vi "HEWH_VESTA_Main.vi"(6 "Vesta is working":refnum<vi>, 8 "error in":errorcluster, 11 "Message Queues out":T2) -> (0 "error out":errorcluster)   [LabVIEW 2023]
uses:
  Tenney/support/Message Queue/All Message Queues.ctl
  Tenney/support/Message Queue/Message Cluster.ctl
  Drivers/Resideo Gas Valve/Type Definitions/Vesta Info.ctl
  Drivers/Resideo Gas Valve/Type Definitions/Temperature Control.ctl
  FVIR and LDO/support/Message Queue/Enqueue Message (Single).vi
  FVIR and LDO/support/Message Queue/Message Queue.lvlib
  Tenney/support/Message Queue/Tenney Message Queue.lvlib
panel:
  out "Vesta Data Output":T1
  out "Debug":string[](array[string])
  in  "Debug":bool
  out "Loop Count":i32
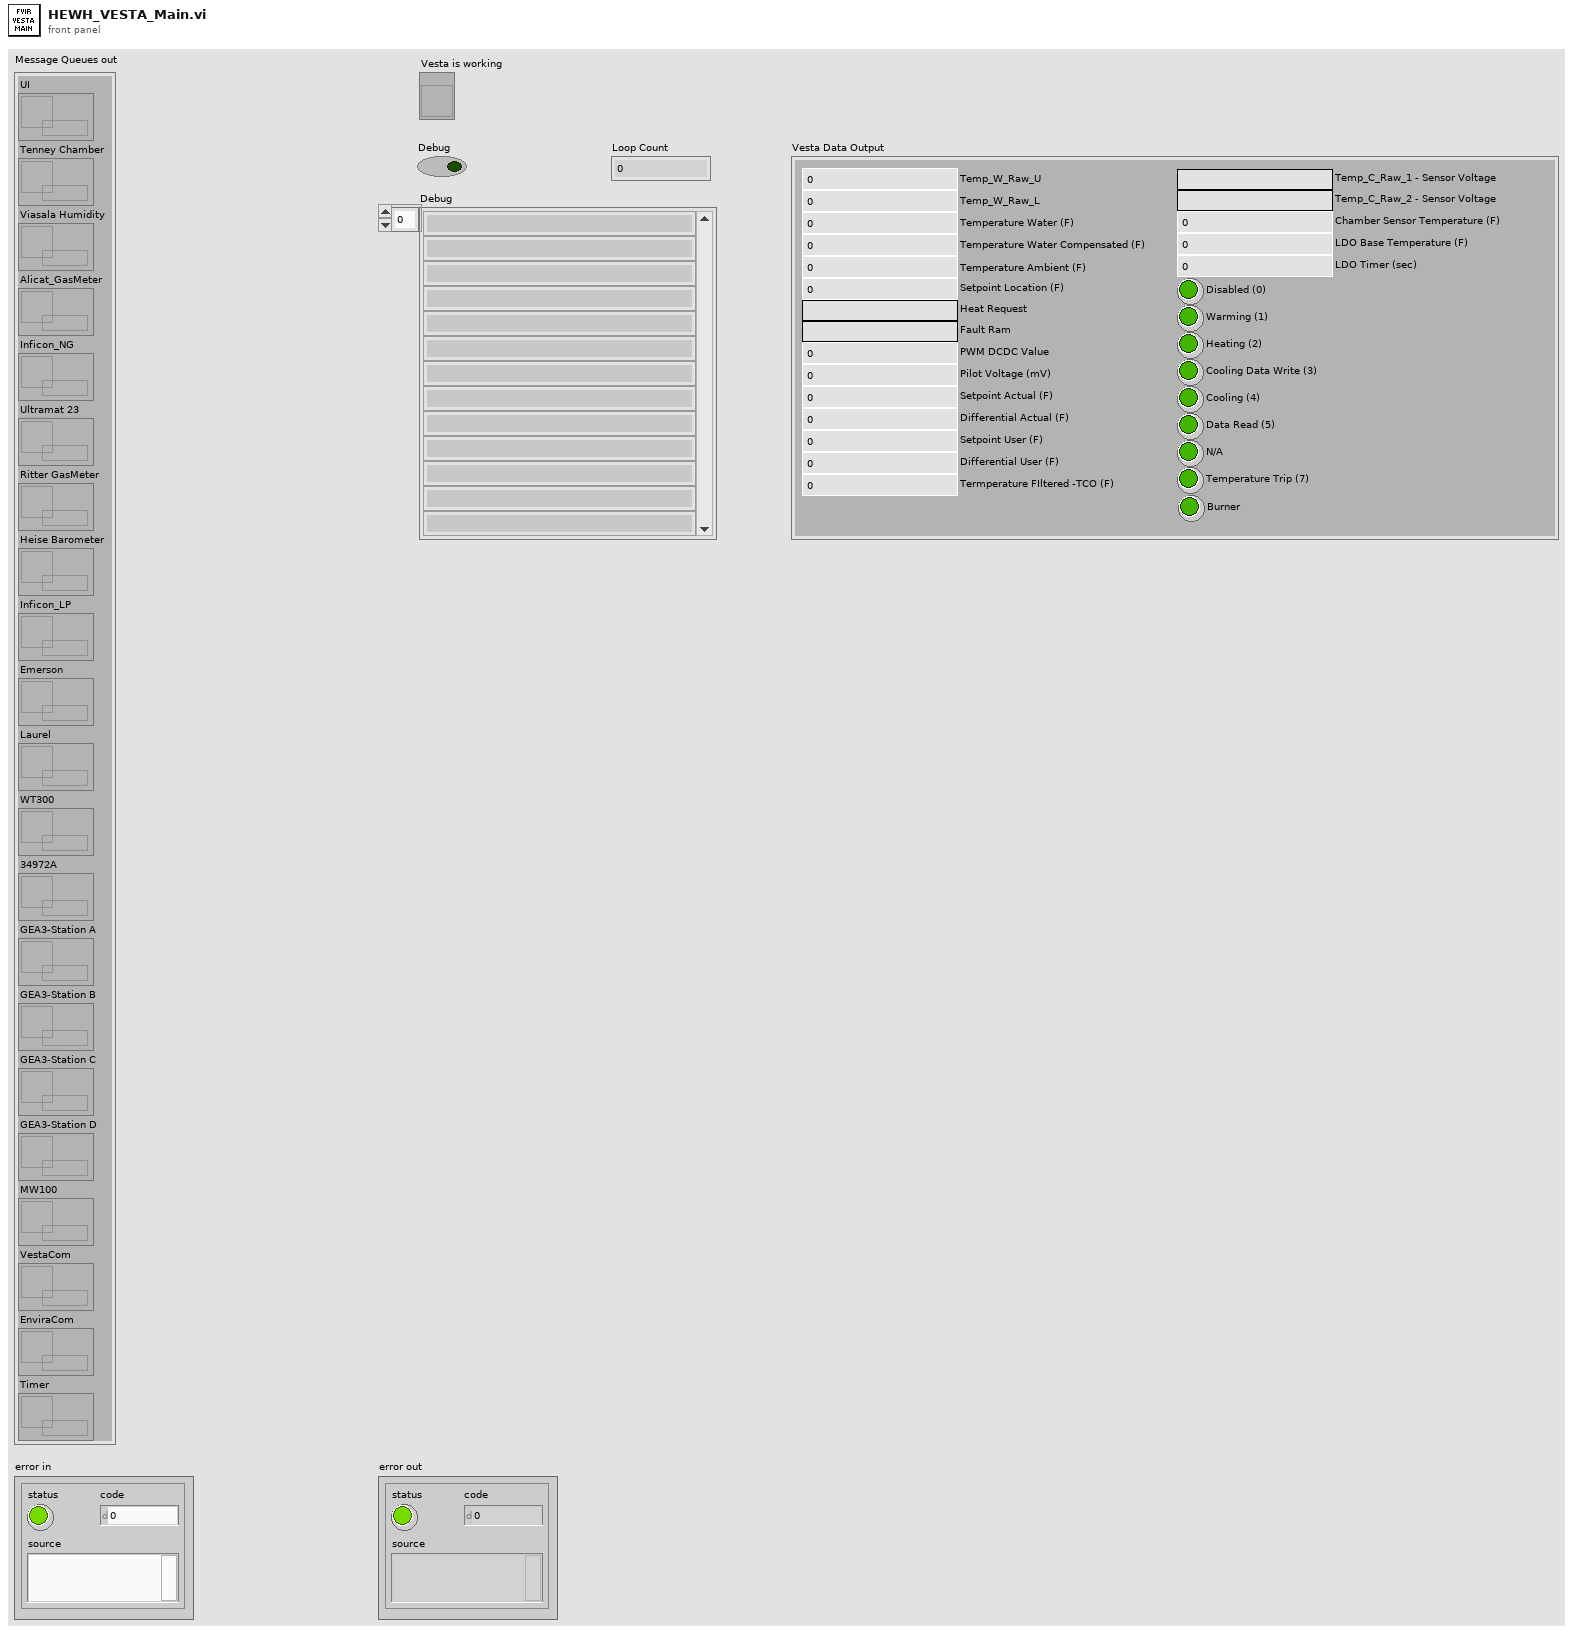
[diagram p1: front panel]
types:
  T1 = typedef "Vesta Info.ctl" = cluster{"Temp_W_Raw_U":u16, "Temp_W_Raw_L":u16, "Temperature Water (F)":dbl, "Temperature Water Compensated (F)":dbl, "Temperature Ambient (F)":dbl, "Setpoint Location (F)":dbl, "Heat Request":string, "Fault Ram":string, "PWM DCDC Value":u16, "Pilot Voltage (mV)":dbl, "Setpoint Actual (F)":dbl, "Differential Actual (F)":dbl, "Setpoint User (F)":dbl, "Differential User (F)":dbl, "Termperature FIltered -TCO (F)":dbl, "Temp_C_Raw_1 - Sensor Voltage":string, "Temp_C_Raw_2 - Sensor Voltage":string, "Chamber Sensor Temperature (F)":dbl, "LDO Base Temperature (F)":dbl, "LDO Timer (sec)":i16, "Disabled (0)":bool, "Warming (1)":bool, "Heating (2)":bool, "Cooling Data Write (3)":bool, "Cooling (4)":bool, "Data Read (5)":bool, "N/A":bool, "Temperature Trip (7)":bool, "Burner":bool}
  T2 = typedef "Tenney Message Queue.lvlib/All Message Queues.ctl" = cluster{"UI":refnum<queue>, "Tenney Chamber":refnum<queue>, "Viasala Humidity":refnum<queue>, "Alicat_GasMeter":refnum<queue>, "Inficon_NG":refnum<queue>, "Ultramat 23":refnum<queue>, "Ritter GasMeter":refnum<queue>, "Heise Barometer":refnum<queue>, "Inficon_LP":refnum<queue>, "Emerson":refnum<queue>, "Laurel":refnum<queue>, "WT300":refnum<queue>, "34972A":refnum<queue>, "GEA3-Station A":refnum<queue>, "GEA3-Station B":refnum<queue>, "GEA3-Station C":refnum<queue>, "GEA3-Station D":refnum<queue>, "MW100":refnum<queue>, "VestaCom":refnum<queue>, "EnviraCom":refnum<queue>, "Timer":refnum<queue>}
  T3 = typedef "Temperature Control.ctl" = cluster{"Water Heater Temp (°F)":u16, "Differential  (°F)":dbl}
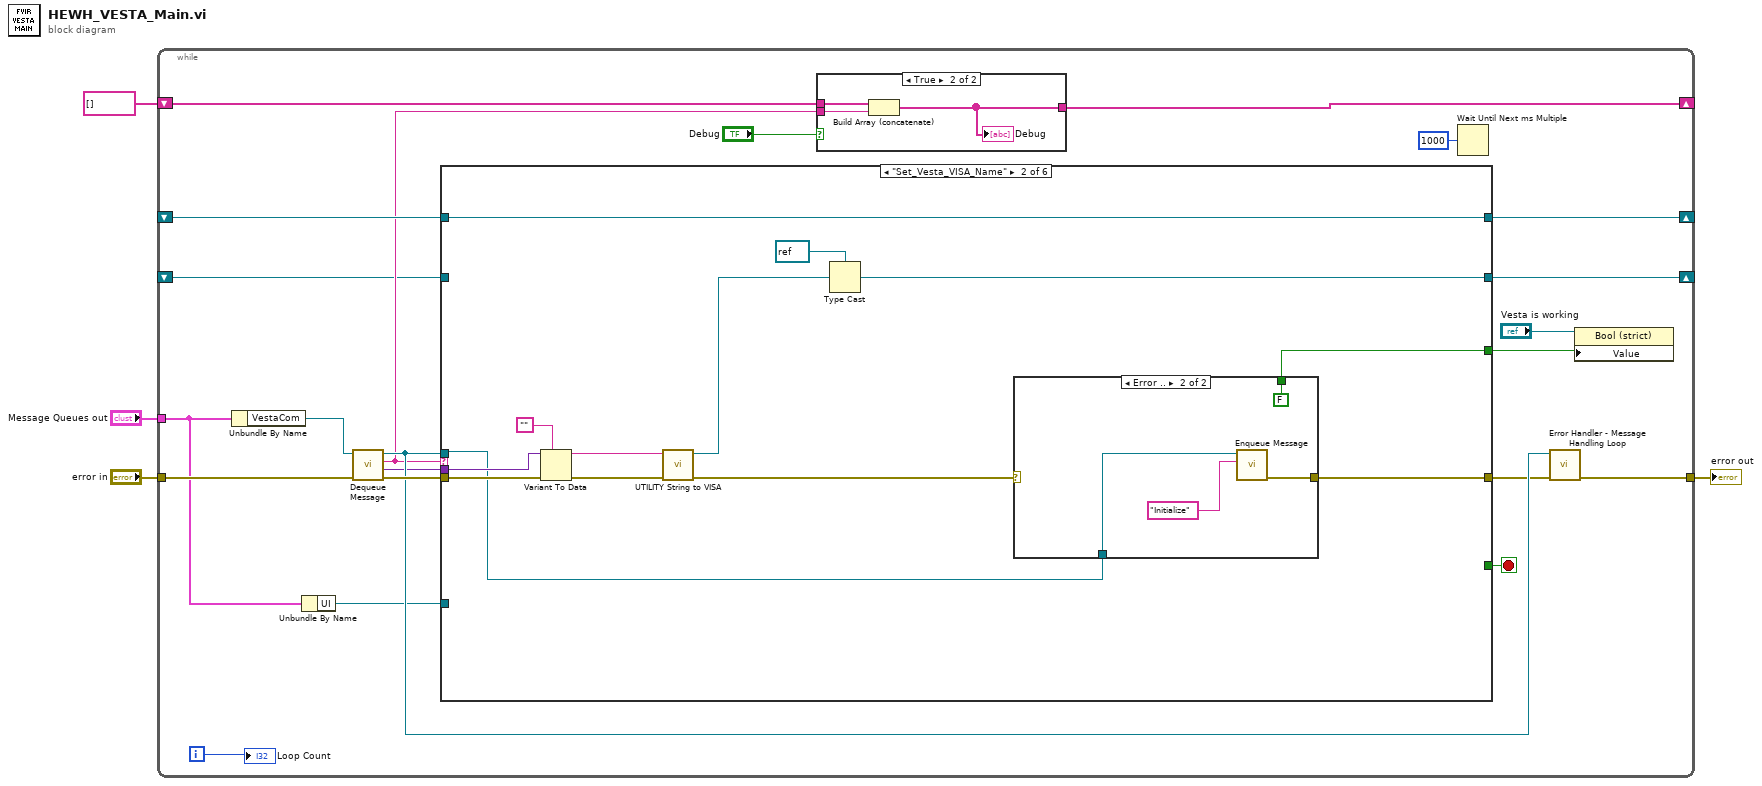
[diagram p0: block diagram]
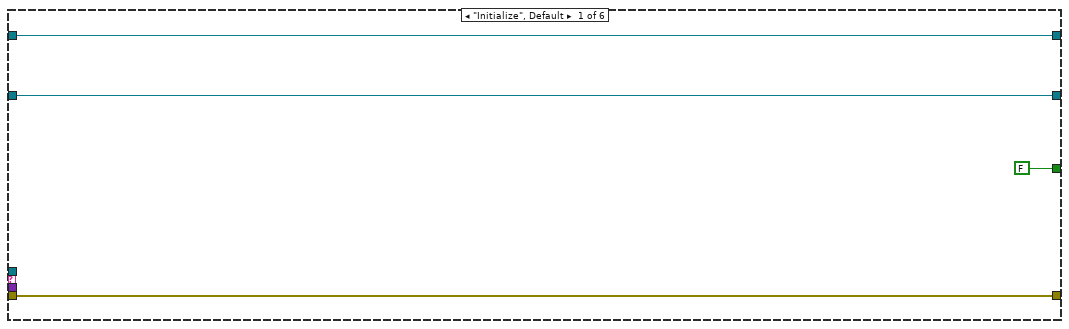
[diagram p3: hidden frame]
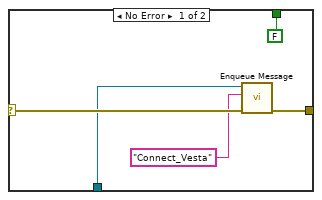
[diagram p4: hidden frame]
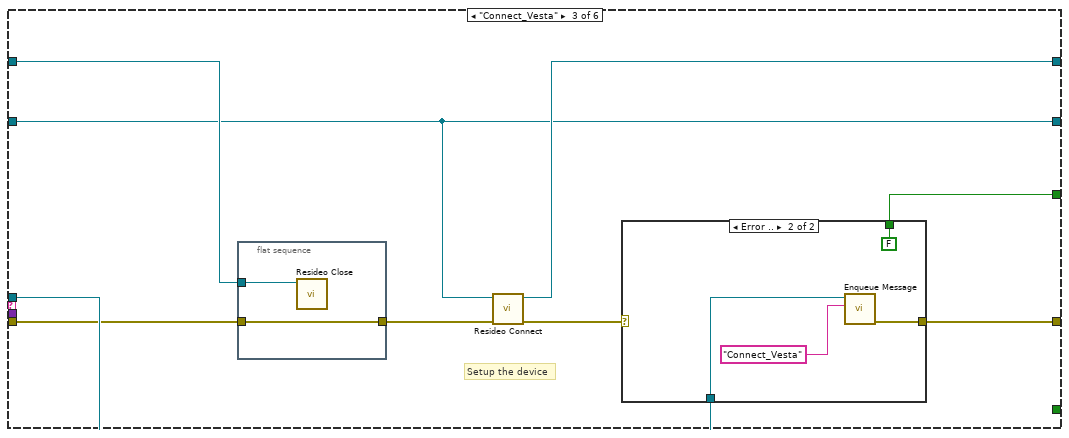
[diagram p5: hidden frame]
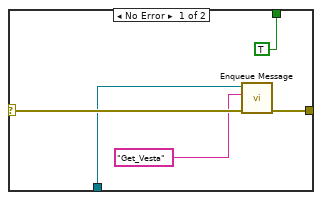
[diagram p6: hidden frame]
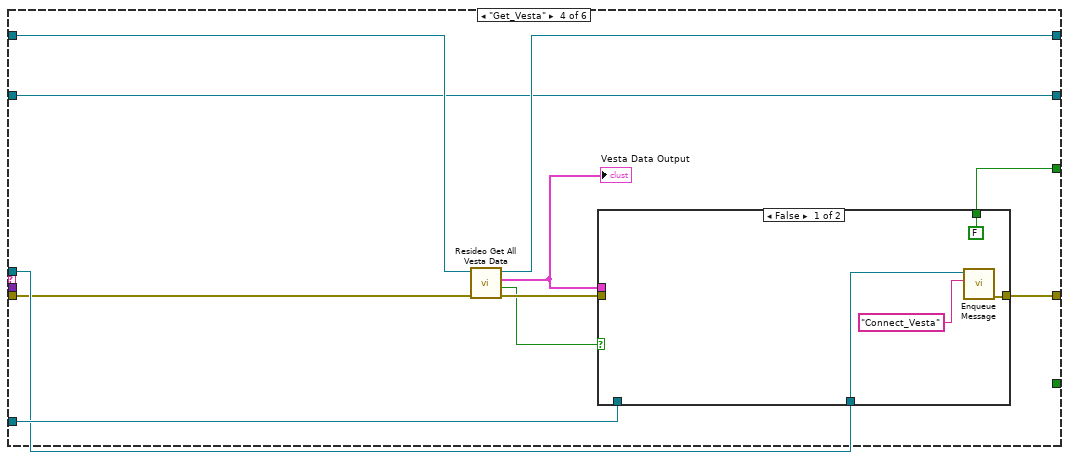
[diagram p7: hidden frame]
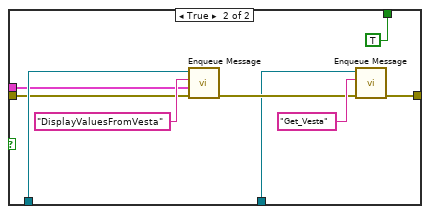
[diagram p8: hidden frame]
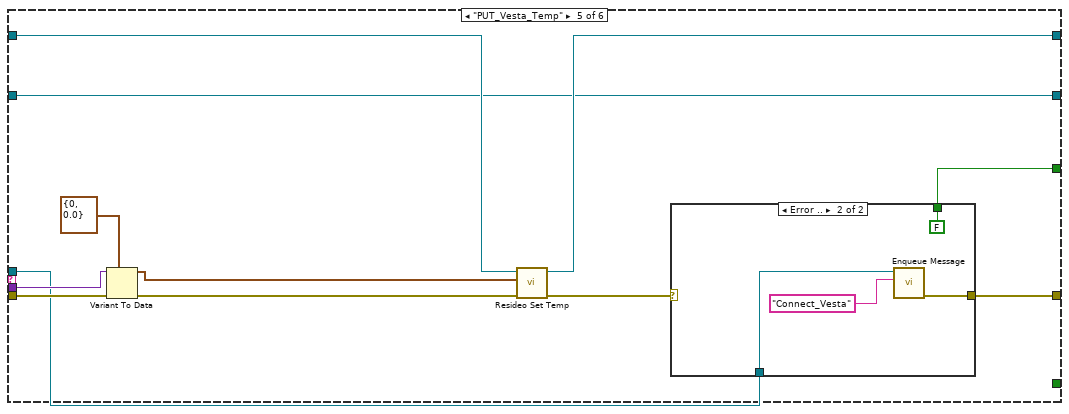
[diagram p9: hidden frame]
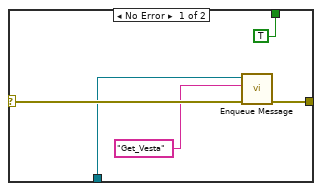
[diagram p10: hidden frame]
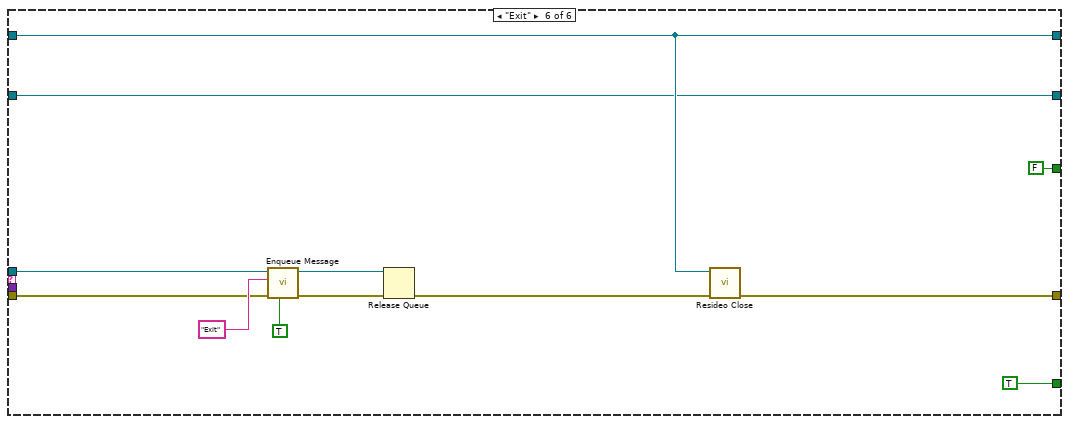
[diagram p11: hidden frame]
diagram:
  n1 = while {
    tunnel: "Message Queues out" -> [w18]
    tunnel: "error in" -> [w25]
    tunnel: [w21] -> w3
    shift-right: [w16] -> _
    shift-left: _ -> [w15]
    shift-right: [w10] -> _
    shift-left: string[] [] -> [w11]
    shift-right: [w8] -> _
    shift-left: _ -> [w7]
    i -> [w14]
    stop <- w23 stop-if-true
    n2 = Unbundle By Name(w18) -> ("VestaCom"=w26:refnum<queue>)
    n3 = Unbundle By Name(w18) -> ("UI"=w17:refnum<queue>)
    n4 = call "Dequeue Message.vi"("error in (no error)"=w25, "Message Queue"=w26) -> ("error out"=w24:errorcluster, "Message Data"=w13:variant, "Message"=w9:string, "dup Message Queue"=w22:refnum<queue>)  [unwired: 6 in]
    n5 = case shown="\"Set_Vesta_VISA_Name\"" w9 {
      tunnel: w24 -> [w33 w45 w60 w84 w112 w130]
      tunnel: [w33 w40 w62 w86 w104 w127] -> w20
      tunnel: [_ _ _ _ _ TRUE] -> w23
      tunnel: w22 -> [_ w39 w63 w85 w103 w125]
      tunnel: w17 -> [_ _ _ w87 _ _]
      tunnel: [w34 w47 w64 w82 w107 w126] -> w16
      tunnel: w15 -> [w34 w47 w61 w83 w108 w126]
      tunnel: w13 -> [_ w44 _ _ w111 _]
      tunnel: [w32 w35 w57 w78 w102 w123] -> w8
      tunnel: w7 -> [w32 _ w57 w78 w102 w123]
      tunnel: [FALSE ("Value") w38 w58 w77 w101 FALSE ("Value")] -> w5
      frame "Initialize", Default {
      }
      frame "Set_Vesta_VISA_Name" {
        n6 = Variant To Data(error in=w45, type="", Variant=w44) -> (data=w42:string, error out=w43:errorcluster)
        n7 = call "UTILITY String to VISA.vi"("error in (no error)"=w43, "VISA Name"=w42) -> ("error out"=w41:errorcluster, "VISA resource name out"=w37:refnum<visa-resource-name>)  [unwired: 8 in]
        n8 = Type Cast(type=refnum<visa-resource-name> refnum ("VISA Refnum in"), x=w37) -> (*(type *) &x=w35:refnum<visa-resource-name>)
        n9 = case shown="Error .." w41 {
          selector: w41 -> [w52 _]
          tunnel: w39 -> [w51 w56]
          tunnel: [w49 w54] -> w40
          tunnel: [FALSE ("Value") FALSE ("Value")] -> w38
          frame No Error {
            n10 = call-poly "Enqueue Message.vi"("error in (no error)"=w52, "Message"="Connect_Vesta", "Message Queue"=w51) -> ("error out"=w49:errorcluster)  [unwired: 7 in, 1 out]
          }
          frame Error {
            n11 = call-poly "Enqueue Message.vi"("Message"="Initialize", "Message Queue"=w56) -> ("error out"=w54:errorcluster)  [unwired: 8 in, 1 out]
          }
        }
      }
      frame "Connect_Vesta" {
        # "Setup the device"
        n12 = flat-sequence {
          tunnel: w61 -> [w67]
          tunnel: w60 -> [w66]
          tunnel: [w66] -> w59
          frame #0 {
            n13 = call "Resideo Close.vi"("Modbus Master in"=w67) -> ()  [unwired: 10 in, 1 out]
          }
        }
        n14 = call "Resideo Connect.vi"("error in (no error)"=w59, "VISA Refnum in"=w57) -> ("error out"=w65:errorcluster, "Modbus Master out"=w64:refnum<class "Modbus Master.lvclass">)  [unwired: 8 in]
        n15 = case shown="Error .." w65 {
          selector: w65 -> [w72 _]
          tunnel: w63 -> [w71 w76]
          tunnel: [w69 w74] -> w62
          tunnel: [TRUE ("Value") FALSE ("Value")] -> w58
          frame No Error {
            n16 = call-poly "Enqueue Message.vi"("error in (no error)"=w72, "Message"="Get_Vesta", "Message Queue"=w71) -> ("error out"=w69:errorcluster)  [unwired: 7 in, 1 out]
          }
          frame Error {
            n17 = call-poly "Enqueue Message.vi"("Message"="Connect_Vesta", "Message Queue"=w76) -> ("error out"=w74:errorcluster)  [unwired: 8 in, 1 out]
          }
        }
      }
      frame "Get_Vesta" {
        n18 = call "Resideo Get All Vesta Data.vi"("error in (no error)"=w84, "Modbus Master in"=w83) -> ("error out"=w80:errorcluster, "Vesta Is Working"=w79:bool, "Vesta Data Output"=w81:T1, "Modbus Master out"=w82:refnum<class "Modbus Master.lvclass">)  [unwired: 6 in]
        "Vesta Data Output" <- w81
        n19 = case shown="False" w79 {
          tunnel: w87 -> [_ w99]
          tunnel: [w90 w96] -> w86
          tunnel: w85 -> [w89 w95]
          tunnel: w80 -> [_ w94]
          tunnel: w81 -> [_ w93]
          tunnel: [FALSE ("Value") TRUE ("Value")] -> w77
          frame False {
            n20 = call-poly "Enqueue Message.vi"("Message"="Connect_Vesta", "Message Queue"=w89) -> ("error out"=w90:errorcluster)  [unwired: 8 in, 1 out]
          }
          frame True {
            n21 = call-poly "Enqueue Message.vi"("error in (no error)"=w94, "Message Data"=w93, "Message"="DisplayValuesFromVesta", "Message Queue"=w99) -> ("error out"=w97:errorcluster)  [unwired: 6 in, 1 out]
            n22 = call-poly "Enqueue Message.vi"("error in (no error)"=w97, "Message"="Get_Vesta", "Message Queue"=w95) -> ("error out"=w96:errorcluster)  [unwired: 7 in, 1 out]
          }
        }
      }
      frame "PUT_Vesta_Temp" {
        n23 = Variant To Data(error in=w112, type=T3 {"Water Heater Temp (°F)"=0, "Differential  (°F)"=0.0} ("Temperature Parameters"), Variant=w111) -> (data=w109:T3, error out=w110:errorcluster)
        n24 = call "Resideo Set Temp.vi"("error in (no error)"=w110, "Vesta Data"=w109, "Modbus Master in"=w108) -> ("error out"=w105:errorcluster, "Modbus Master out"=w107:refnum<class "Modbus Master.lvclass">)  [unwired: 7 in]
        n25 = case shown="Error .." w105 {
          selector: w105 -> [w117 _]
          tunnel: w103 -> [w116 w121]
          tunnel: [w114 w119] -> w104
          tunnel: [TRUE ("Value") FALSE ("Value")] -> w101
          frame No Error {
            n26 = call-poly "Enqueue Message.vi"("error in (no error)"=w117, "Message"="Get_Vesta", "Message Queue"=w116) -> ("error out"=w114:errorcluster)  [unwired: 7 in, 1 out]
          }
          frame Error {
            n27 = call-poly "Enqueue Message.vi"("Message"="Connect_Vesta", "Message Queue"=w121) -> ("error out"=w119:errorcluster)  [unwired: 8 in, 1 out]
          }
        }
      }
      frame "Exit" {
        n28 = call-poly "Enqueue Message.vi"("Priority Message? (F)"=TRUE, "error in (no error)"=w130, "Message"="Exit", "Message Queue"=w125) -> ("error out"=w129:errorcluster, "dup Message Queue"=w124:refnum<queue>)  [unwired: 6 in]
        n29 = Release Queue(queue=w124, error in (no error)=w129) -> (error out=w128:errorcluster)  [unwired: 1 in, 2 out]
        n30 = call "Resideo Close.vi"("error in (no error)"=w128, "Modbus Master in"=w126) -> ("error out"=w127:errorcluster)  [unwired: 9 in]
      }
    }
    n31 = case shown="True" "Debug" {
      tunnel: w9 -> [_ w30]
      tunnel: w11 -> [w27 w29]
      tunnel: [w27 w28] -> w10
      frame False {
      }
      frame True {
        n32 = Build Array (concatenate)(w29, w30) -> (w28:string[])
        "Debug" <- w28
      }
    }
    n33 = Wait Until Next ms Multiple(millisecond multiple=u32 1000) -> ()  [unwired: 1 out]
    n34 = call "Error Handler - Message Handling Loop.vi"("error in (no error)"=w20, "Message Queue"=w22) -> ("dup error in"=w21:errorcluster)  [unwired: 8 in, 1 out]
    n35 = property class="Bool (strict)"(reference="Vesta is working", "Value"=w5) -> ()  [unwired: 1 in, 2 out]
    "Loop Count" <- w14
  }
  "error out" <- w3
